vi "Get Document Source.vi"(8 "Error In":errorcluster, 11 "WebView in":refnum<class "WebView.lvclass">) -> (0 "Error Out":errorcluster, 2 "Document Source":string, 3 "WebView out":refnum<class "WebView.lvclass">)   [LabVIEW 2024, in "WebView.lvclass"]
uses:
  WebView.lvclass
  WebView.lvclass/WebView.ctl
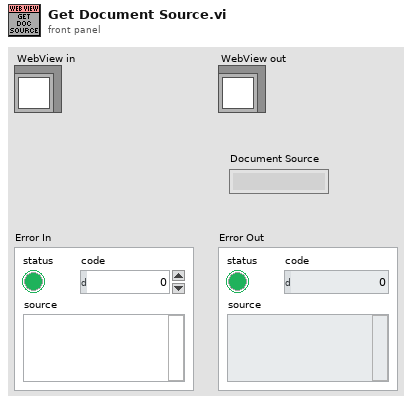
[diagram p1: front panel]
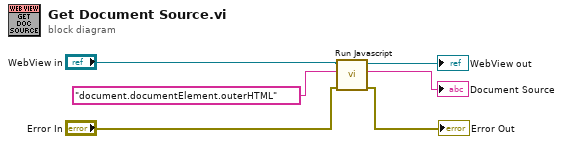
[diagram p0: block diagram]
diagram:
  n1 = call "Run Javascript.vi"("Error In"="Error In", "Javascript in"="document.documentElement.outerHTML" ("javaScript"), "WebView in"="WebView in") -> ("Error Out"=→"Error Out":errorcluster, "Result out"=→"Document Source":string, "WebView out"=→"WebView out":refnum<class "WebView.lvclass">)  [unwired: 6 in]
